vi "写入缺试剂参数.vi"(8 "error in (no error)":errorcluster, 9 "光强阈值":u16[](array[numeric]), 10 "缺试剂类型":u8[](array[numeric]), 11 "MB session in":refnum<class "MB_Master.lvclass">) -> (0 "error out":errorcluster, 3 "MB session out":refnum<class "MB_Master.lvclass">)   [LabVIEW 2016]
uses:
  <vilib>/Plasmionique/MB Master/MB_Master/MB_Master.lvclass
  <vilib>/Plasmionique/MB Master/MB_Master_Serial/MB_Master_Serial.lvclass
  D:/Program Files (x86)/National Instruments/LabVIEW 2016/vi.lib/Plasmionique/MB Master/MB_Master/MB_Master.lvclass
  <vilib>/Plasmionique/MB Master/MB Master.lvlib
panel:
  in  "VISA Resource":refnum<visa-resource-name>
  in  "引用选择":enum16{"MB引用", "自建引用"}(ring)
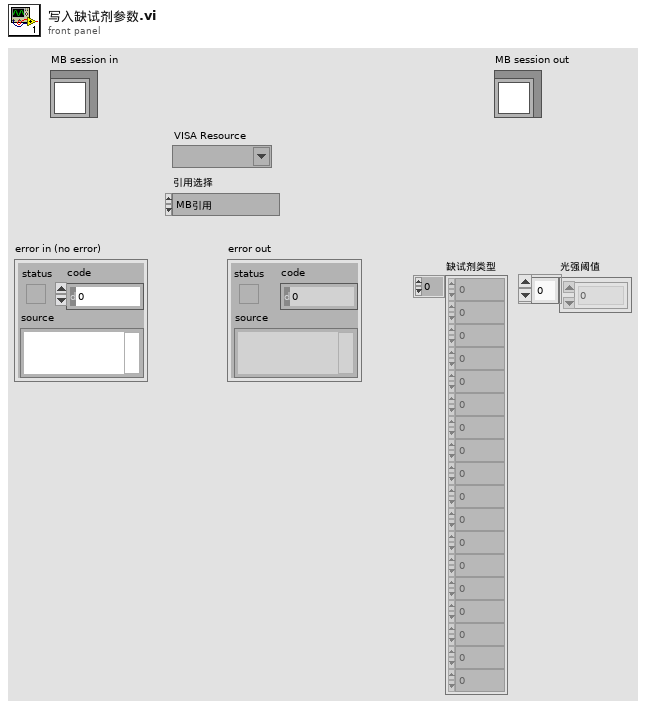
[diagram p1: front panel]
types:
  T1 = cluster{"baud rate (bps)":u32, "stop bits":u16, "parity":u16, "flow control":u16, "timeout":u32, "retries":i32}
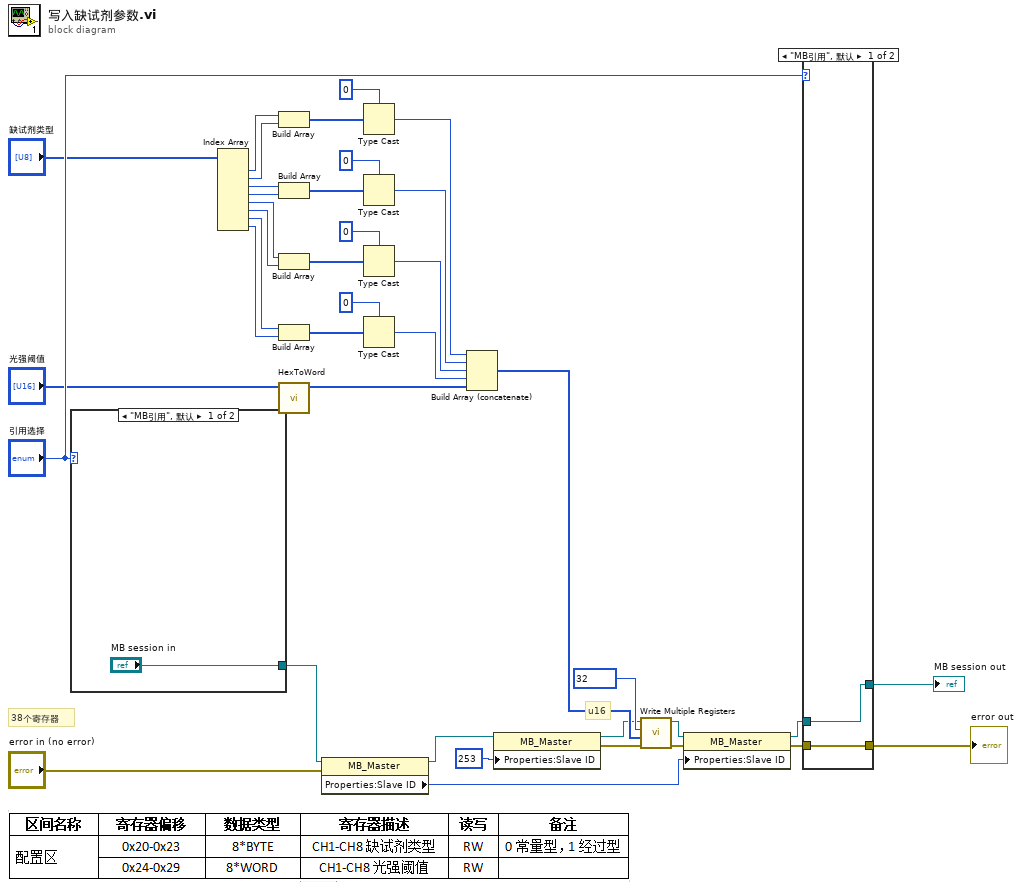
[diagram p0: block diagram]
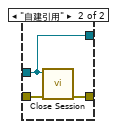
[diagram p2: hidden frame]
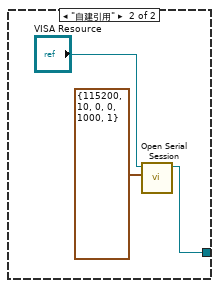
[diagram p3: hidden frame]
diagram:
  # "38个寄存器"
  # "u16"
  n1 = case shown="\"MB引用\", 默认" "引用选择" {
    tunnel: ["MB session in" w43] -> w8
    frame "MB引用", Default {
    }
    frame "自建引用" {
      n2 = call <vilib>:"Open Serial Session.vi"("Serial Config"=T1 {"baud rate (bps)"=115200, "stop bits"=10, "parity"=0, "flow control"=0, "timeout"=1000, "retries"=1}, "VISA Resource"="VISA Resource") -> ("MB_Serial session"=w43:refnum<class "MB_Master_Serial.lvclass">)  [unwired: 8 in, 1 out]
    }
  }
  n3 = Index Array(array="缺试剂类型") -> (element #1=w24:u8, element #2=w23:u8, element #3=w22:u8, element #4=w21:u8, element #5=w18:u8, element #6=w17:u8, element #7=w16:u8, element #8=w15:u8)  [unwired: 8 in]
  n4 = Build Array(w24, w23) -> (w34:u8[])
  n5 = Build Array(w22, w21) -> (w33:u8[])
  n6 = Build Array(w18, w17) -> (w20:u8[])
  n7 = Build Array(w16, w15) -> (w28:u8[])
  n8 = call "HexToWord.vi"("数组"="光强阈值") -> ("WORD"=w11:u16[])  [unwired: 10 in]
  n9 = property class="MB_Master"(reference=w8, error in="error in (no error)") -> (reference out=w6:refnum<class "MB_Master.lvclass">, "Properties:Slave ID"=w1:u8)  [unwired: 1 out]
  n10 = Type Cast(type=u16 0, x=w34) -> (*(type *) &x=w30:u16)
  n11 = Type Cast(type=u16 0, x=w33) -> (*(type *) &x=w29:u16)
  n12 = Type Cast(type=u16 0, x=w20) -> (*(type *) &x=w14:u16)
  n13 = Type Cast(type=u16 0, x=w28) -> (*(type *) &x=w13:u16)
  n14 = Build Array (concatenate)(w30, w29, w14, w13, w11) -> (w31:u16[])
  n15 = property class="MB_Master"(reference=w6, "Properties:Slave ID"=u8 253 ("Slave ID")) -> (reference out=w9:refnum<class "MB_Master.lvclass">, error out=w10:errorcluster)  [unwired: 1 in]
  n16 = call <vilib>:"Write Multiple Registers.vi"("error in (no error)"=w10, "values"=w31, "starting address"=u16 32, "MB session in"=w9) -> ("error out"=w4:errorcluster, "MB session out"=w5:refnum<class "MB_Master.lvclass">)  [unwired: 6 in]
  n17 = property class="MB_Master"(reference=w5, error in=w4, "Properties:Slave ID"=w1) -> (reference out=w3:refnum<class "MB_Master.lvclass">, error out=w2:errorcluster)
  n18 = case shown="\"MB引用\", 默认" "引用选择" {
    tunnel: w3 -> [w44 w46]
    tunnel: w2 -> [w45 w48]
    tunnel: [w45 w47] -> w37
    tunnel: [w44 w46] -> w36
    frame "MB引用", Default {
    }
    frame "自建引用" {
      n19 = call-dynamic "Close Session.vi"("error in (no error)"=w48, "MB session in"=w46) -> ("error out"=w47:errorcluster)  [unwired: 9 in]
    }
  }
  "MB session out" <- w36
  "error out" <- w37
